vi "FindMassResolution_Single.vi"(7 "EnableResDisplay":bool, 10 "BinnedSpectrum":cluster{"m/z Array":dbl[], "Signal":dbl[]}, 11 "GraphRef":refnum<vi>) -> (2 "FWHM":dbl, 3 "Resolution":dbl)   [LabVIEW 2013]
uses:
  <vilib>/Utility/miscctls.llb/LVCursorListTypeDef.ctl
  <vilib>/Utility/miscctls.llb/LVAnnotationListTypeDef.ctl
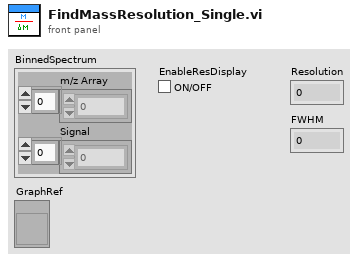
[diagram p1: front panel]
types:
  T1 = typedef "LVAnnotationListTypeDef.ctl" = cluster{"Name":string, "Color":u32, "Style":u8, "Point Style":u8, "Name Visible":bool, "Allow Drag":bool, "Annotation Mode":u32, "Plot":i32, "Index":i32, "Position":cluster{"X":dbl, "Y":dbl}, "X Scale":u32, "Y Scale":u32, "Show Arrow":bool, "Lock Name":bool, "Plot Area":i32, "Label Offset":cluster{"X":dbl, "Y":dbl}}[]
  T2 = typedef "LVCursorListTypeDef.ctl" = cluster{"Name":string, "Color":u32, "Style":u8, "Point Style":u8, "Name Visible":bool, "Allow Drag":bool, "Cursor Mode":u32, "Plot":i32, "Index":i32, "Position":cluster{"X":dbl, "Y":dbl}, "X Scale":u32, "Y Scale":u32, "Watch Plots":i32[], "Watch All Plots":bool, "Plot Area":i32, "Label Offset":cluster{"X":dbl, "Y":dbl}}[]
  T3 = cluster{"Name":string, "Color":u32, "Style":u8, "Point Style":u8, "Name Visible":bool, "Allow Drag":bool, "Annotation Mode":u32, "Plot":i32, "Index":i32, "Position":cluster{"X":dbl, "Y":dbl}, "X Scale":u32, "Y Scale":u32, "Show Arrow":bool, "Lock Name":bool, "Plot Area":i32, "Label Offset":cluster{"X":dbl, "Y":dbl}}
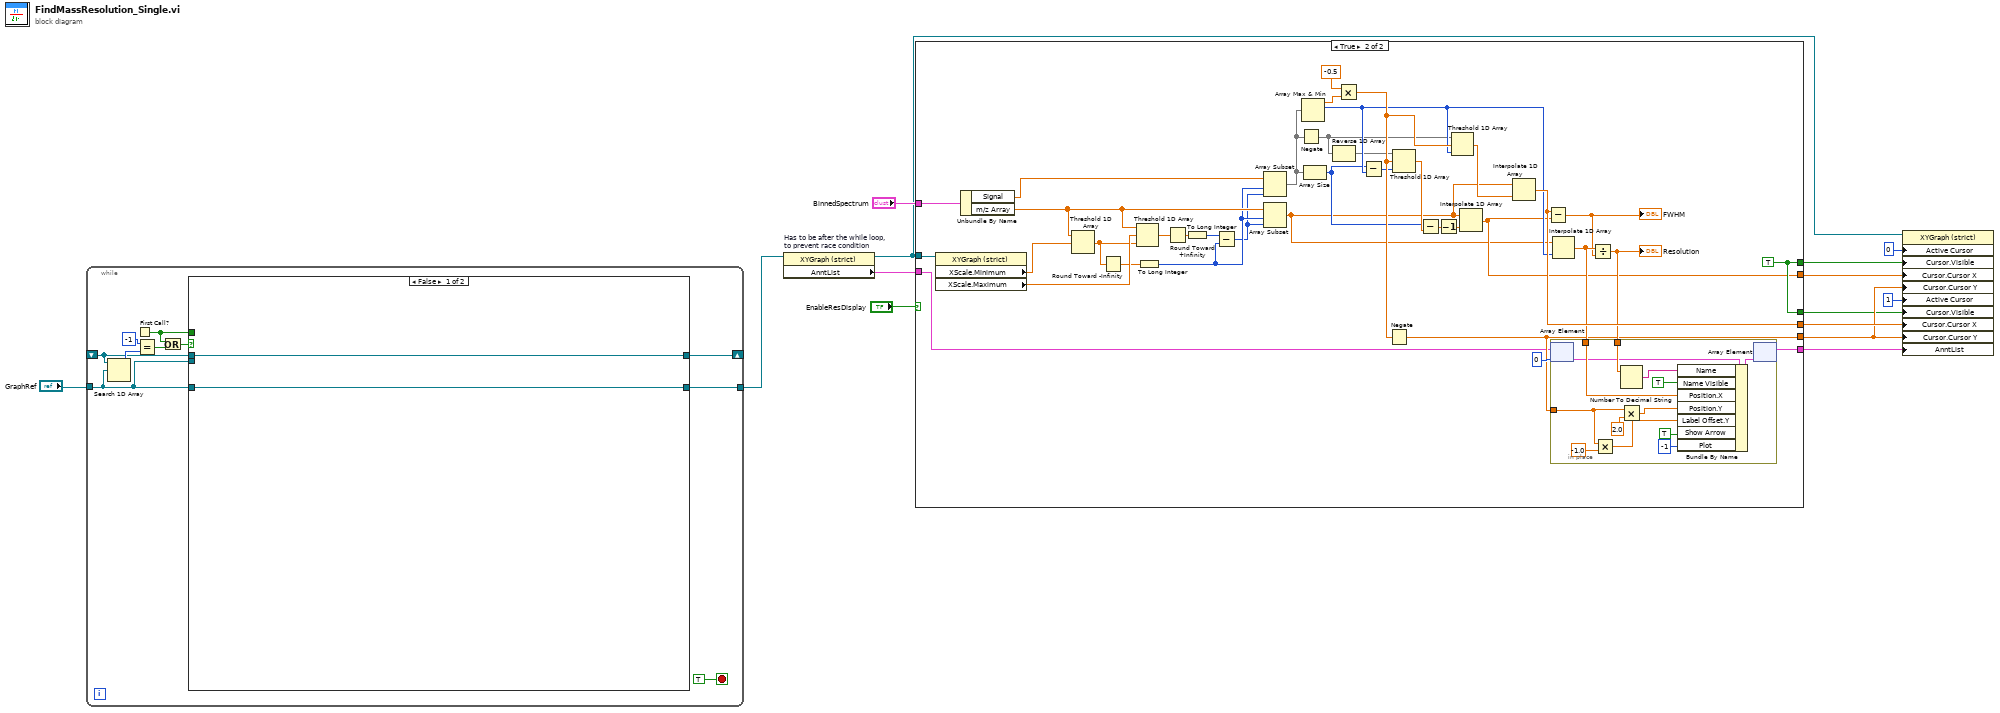
[diagram p0: block diagram]
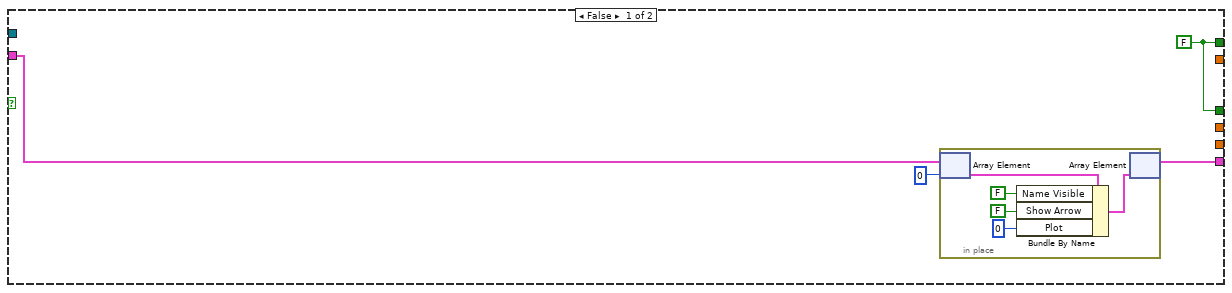
[diagram p2: hidden frame]
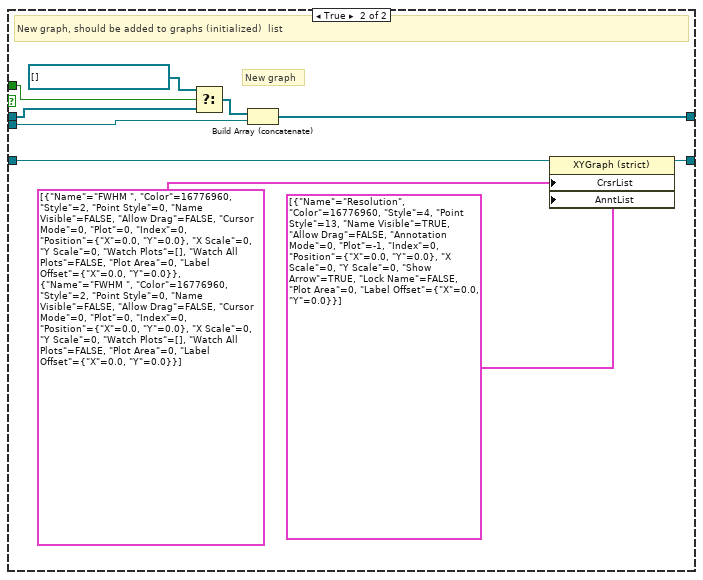
[diagram p3: hidden frame]
diagram:
  n1 = while {
    tunnel: "GraphRef" -> [w21]
    shift-right: [w20] -> _
    shift-left: _ -> [w19]
    tunnel: [w15] -> w1
    stop <- TRUE stop-if-true
    n2 = Search 1D Array(1D array=w19, element=w21) -> (index of element=w23:i32)  [unwired: 1 in]
    n3 = First Call?() -> (First Call?: T/F=w16:bool)
    n4 = Equal?(x=-1, y=w23) -> (x = y?=w22:bool)
    n5 = Or(x=w16, y=w22) -> (x .or. y?=w17:bool)
    n6 = case shown="False" w17 {
      tunnel: w19 -> [w26 w31]
      tunnel: [w26 w36] -> w20
      tunnel: w21 -> [_ w35]
      tunnel: w21 -> [w25 w34]
      tunnel: w16 -> [_ w28]
      tunnel: [w25 w27] -> w15
      frame False {
      }
      frame True {
        # "New graph"
        # "New graph, should be added to graphs (initialized)  list"
        n7 = Select(t=refnum<vi>[] [], s=w28, f=w31) -> (s? t:f=w30:refnum<vi>[])
        n8 = Build Array (concatenate)(w30, w35) -> (w36:refnum<vi>[])
        n9 = property class="XYGraph (strict)"(reference=w34, "CrsrList"=T2 [{"Name"="FWHM ", "Color"=16776960, "Style"=2, "Point Style"=0, "Name Visible"=FALSE, "Allow Drag"=FALSE, "Cursor Mode"=0, "Plot"=0, "Index"=0, "Position"={"X"=0.0, "Y"=0.0}, "X Scale"=0, "Y Scale"=0, "Watch Plots"=[], "Watch All Plots"=FALSE, "Plot Area"=0, "Label Offset"={"X"=0.0, "Y"=0.0}}, {"Name"="FWHM ", "Color"=16776960, "Style"=2, "Point Style"=0, "Name Visible"=FALSE, "Allow Drag"=FALSE, "Cursor Mode"=0, "Plot"=0, "Index"=0, "Position"={"X"=0.0, "Y"=0.0}, "X Scale"=0, "Y Scale"=0, "Watch Plots"=[], "Watch All Plots"=FALSE, "Plot Area"=0, "Label Offset"={"X"=0.0, "Y"=0.0}}] ("Cursor List"), "AnntList"=T1 [{"Name"="Resolution", "Color"=16776960, "Style"=4, "Point Style"=13, "Name Visible"=TRUE, "Allow Drag"=FALSE, "Annotation Mode"=0, "Plot"=-1, "Index"=0, "Position"={"X"=0.0, "Y"=0.0}, "X Scale"=0, "Y Scale"=0, "Show Arrow"=TRUE, "Lock Name"=FALSE, "Plot Area"=0, "Label Offset"={"X"=0.0, "Y"=0.0}}] ("Annotation List")) -> (reference out=w27:refnum<vi>)  [unwired: 1 in, 1 out]
      }
    }
  }
  n10 = property on="Has to be after the while loop,\nto prevent race condition" class="XYGraph (strict)"(reference=w1) -> (reference out=w2:refnum<vi>, "AnntList"=w3:T1)  [unwired: 1 in, 1 out]
  n11 = case shown="True" "EnableResDisplay" {
    tunnel: "BinnedSpectrum" -> [_ w82]
    tunnel: w2 -> [_ w81]
    tunnel: [_ w53] -> w12
    tunnel: [_ w71] -> w11
    tunnel: [_ w54] -> w10
    tunnel: [w38 w59] -> w6
    tunnel: [w40 w58] -> w9
    tunnel: [w40 w58] -> w8
    tunnel: w3 -> [w37 w47]
    frame False {
      w40 = FALSE
      n12 = in-place {
        n13 = in-place-array #1(w37, 0) -> (w43:T3)
        n14 = Bundle By Name(cluster=w43, "Name Visible"=FALSE, "Show Arrow"=FALSE, "Plot"=0) -> (w45:T3)
        n15 = in-place-array #1(w45) -> (w38:T1)  [unwired: 1 out]
      }
    }
    frame True {
      w58 = TRUE
      n16 = property class="XYGraph (strict)"(reference=w81) -> ("XScale.Minimum"=w80:dbl, "XScale.Maximum"=w79:dbl)  [unwired: 1 in, 2 out]
      n17 = Unbundle By Name(w82) -> ("Signal"=w70:dbl[], "m/z Array"=w66:dbl[])
      n18 = Threshold 1D Array(2:w80, 3:w66) -> (0:w74:dbl)  [unwired: 1 in]
      n19 = Round Toward -Infinity(1:w74) -> (0:w76:dbl)
      n20 = Threshold 1D Array(1:w74, 2:w79, 3:w66) -> (0:w78:dbl)
      n21 = To Long Integer(number=w76) -> (32bit integer=w65:i32)
      n22 = Round Toward +Infinity(x=w78) -> (ceil(x): smallest int >= x=w77:dbl)
      n23 = To Long Integer(number=w77) -> (32bit integer=w75:i32)
      n24 = Subtract(x=w75, y=w65) -> (x-y=w64:i32)
      n25 = Array Subset(array=w70, index=w65, length=w64) -> (w57:dbl[])
      n26 = Array Subset(array=w66, index=w65, length=w64) -> (w50:dbl[])
      n27 = Negate(x=w57) -> (-x=w48:dbl[])
      n28 = Array Max & Min(array=w57) -> (max value=w73:dbl, max index (indices)=w55:i32)  [unwired: 2 out]
      n29 = Array Size(array=w57) -> (size(s)=w51:i32)
      n30 = Reverse 1D Array(array=w48) -> (reversed array=w49:dbl[])
      n31 = Multiply(x=-0.5, y=w73) -> (x*y=w61:dbl)
      n32 = Subtract(x=w51, y=w55) -> (x-y=w56:i32)
      n33 = Negate(x=w61) -> (-x=w54:dbl)
      n34 = Threshold 1D Array(1:w56, 2:w61, 3:w49) -> (0:w62:dbl)
      n35 = Subtract(x=w51, y=w62) -> (x-y=w52:dbl)
      n36 = Decrement(x=w52) -> (x-1=w46:dbl)
      n37 = Threshold 1D Array(1:w55, 2:w61, 3:w48) -> (0:w63:dbl)
      n38 = Interpolate 1D Array(1:w46, 2:w50) -> (0:w53:dbl)
      n39 = Interpolate 1D Array(1:w63, 2:w50) -> (0:w71:dbl)
      n40 = Subtract(x=w71, y=w53) -> (x-y=w67:dbl)
      "FWHM" <- w67
      n41 = Interpolate 1D Array(1:w55, 2:w50) -> (0:w69:dbl)
      n42 = Divide(x=w69, y=w67) -> (x/y=w60:dbl)
      "Resolution" <- w60
      n43 = in-place {
        in-place-border: w69 -> [w93]
        in-place-border: w54 -> [w87]
        in-place-border: w60 -> [w91]
        n44 = in-place-array #2(w47, 0) -> (w85:T3)
        n45 = Multiply(x=w87, y=-1.0) -> (x*y=w90:dbl)
        n46 = Number To Decimal String(number=w91) -> (decimal integer string=w92:string)  [unwired: 1 in]
        n47 = Multiply(x=w87, y=2.0) -> (x*y=w86:dbl)
        n48 = Bundle By Name(cluster=w85, "Name"=w92, "Name Visible"=TRUE, "Position.X"=w93, "Position.Y"=w86, "Label Offset.Y"=w90, "Show Arrow"=TRUE, "Plot"=-1) -> (w95:T3)
        n49 = in-place-array #2(w95) -> (w59:T1)  [unwired: 1 out]
      }
    }
  }
  n50 = property class="XYGraph (strict)"(reference=w2, "Active Cursor"=u32 0, "Cursor.Visible"=w9, "Cursor.Cursor X"=w12, "Cursor.Cursor Y"=w10, "Active Cursor"=u32 1, "Cursor.Visible"=w8, "Cursor.Cursor X"=w11, "Cursor.Cursor Y"=w10, "AnntList"=w6) -> ()  [unwired: 1 in, 2 out]
